vi "Set ControlValue (U32).vi"(8 "Error In":errorcluster caption="エラー入力", 9 "Value":u32, 10 "Control Name":string, 11 "VI refnum in":refnum<vi>) -> (0 "Error Out":errorcluster caption="エラー出力", 3 "VI refnum out":refnum<vi>)   [LabVIEW 2020]
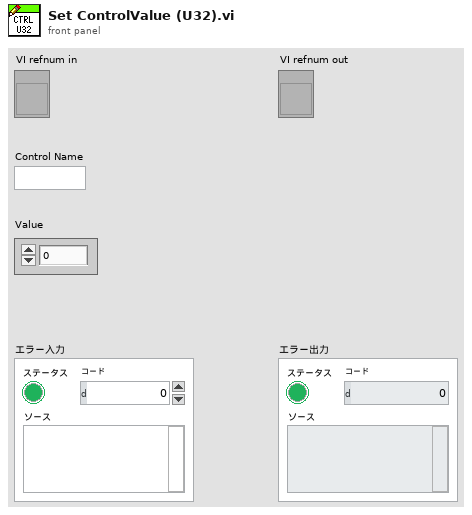
[diagram p1: front panel]
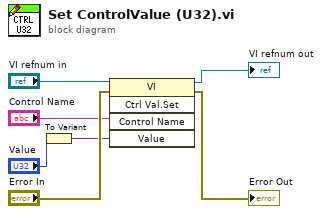
[diagram p0: block diagram]
diagram:
  n1 = To Variant(anything="Value") -> (Variant=w1:variant)
  n2 = invoke class="VI" method="Ctrl Val.Set"(reference="VI refnum in", error in="Error In", "Control Name"="Control Name", "Value"=w1) -> (reference out=→"VI refnum out":refnum<vi>, error out=→"Error Out":errorcluster)  [unwired: 1 in, 3 out]
